vi "Actor Core.vi"(8 "error in":errorcluster, 11 "Launch IMAQ Display in":refnum<class "HIJ Vision Application.lvclass">) -> (0 "error out":errorcluster={"status"=FALSE, "code"=0, "source"="Actor Framework.lvlib:Actor.lvclass:Launch Nested Actor.vi<APPEND>\n\n<b>Complete call chain:</b>\r\n     Actor Framework.lvlib:Actor.lvclass:Launch Nested Actor.vi\r\n     Launch HIJ FileViewer.lvlib:Launch File Viewer.lvclass:Actor Core.vi"}, 3 "Actor out":refnum<class "Actor.lvclass">)   [LabVIEW 2014, in "HIJ Vision Application.lvlib" / "HIJ Vision Application.lvclass"]
doc: "(<B>Filename</B>: Actor Framework.lvlib:Actor.lvclass:Actor Core.vi)\n\nReceives messages to the actor, reacts to them, and initiates any error handling that may shut the actor down.\n\nDescendant classes may override this VI to append parallel tasks for the actor to complete while it handles messages. Overrides use the Call Parent Method node."
uses:
  HIJ Vision Application.lvclass
  <vilib>/ActorFramework/Actor/Actor.lvclass
  <vilib>/ActorFramework/Message Enqueuer/Message Priority.ctl
  HIJ Vision Application Messages/New Results Msg/New Results Msg.lvclass
  HIJ Vision Application.lvclass/HIJ Vision Application.ctl
  Display Actors/HIJ Vision Display/HIJ Vision Display/HIJ Vision Display.lvclass/HIJ Vision Display.ctl
  Analyze/Analyze Actor/Analyze Actor/Analyze Actor.lvclass/Analyze Actor.ctl
  <vilib>/ActorFramework/Actor/Actor.lvclass/Actor.ctl
  <vilib>/ActorFramework/Message Enqueuer/Message Enqueuer.lvclass/Message Enqueuer.ctl
  Display Actors/HIJ Vision Display/HIJ Vision Display Messages/Write Analyze Actor Msg/Write Analyze Enq Msg.lvclass/Write Analyze Enq Msg.ctl
  Shared Code/Viewable Actor/ViewableActor Messages/Insert Into SubPanel Msg/Insert Into SubPanel Msg.lvclass/Insert Into SubPanel Msg.ctl
  Display Actors/HIJ Vision Display/HIJ Vision Display/Read My New Results Msg.vi
  Display Actors/HIJ Vision Display/HIJ Vision Display/Write Publish Analyze Results Msg.vi
  Analyze/Analyze Actor/Analyze Actor/Write Analyze Objects.vi
  Analyze/Analyze Actor/Analyze Actor/Write Publish Analyze Results Msg.vi
  Analyze/Analyze Actor/Analyze Actor/Write Destination.vi
  <vilib>/ActorFramework/Message Enqueuer/Init from Existing Queue.vi
  <vilib>/ActorFramework/Message Enqueuer/Enqueue.vi
  <vilib>/ActorFramework/Message Priority Queue/Priority Enqueue.vi
  Display Actors/HIJ Vision Display/HIJ Vision Display Messages/New Results Msg/New Results Msg.lvclass
  <vilib>/ActorFramework/Message Enqueuer/Message Enqueuer.lvclass
  HIJ Vision Application Messages/After Launch Init Msg/After Launch Init Msg.lvclass
  Display Actors/HIJ Vision Display/HIJ Vision Display Messages/Write Analyze Actor Msg/Write Analyze Enq Msg.lvclass
  Shared Code/Viewable Actor/ViewableActor Messages/Insert Into SubPanel Msg/Insert Into SubPanel Msg.lvclass
  Shared Code/Viewable Actor/ViewableActor/ViewableActor.lvclass
  Display Actors/HIJ Vision Display/HIJ Vision Display/HIJ Vision Display.lvclass
  Analyze/Analyze Actor/Analyze Actor/Analyze Actor.lvclass
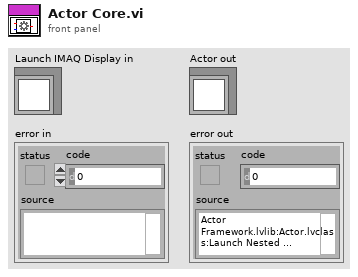
[diagram p1: front panel]
types:
  T1 = typedef "Actor Framework.lvlib/Message Enqueuer.lvclass/Message Priority.ctl" = enum16{"Low", "Normal", "High"}
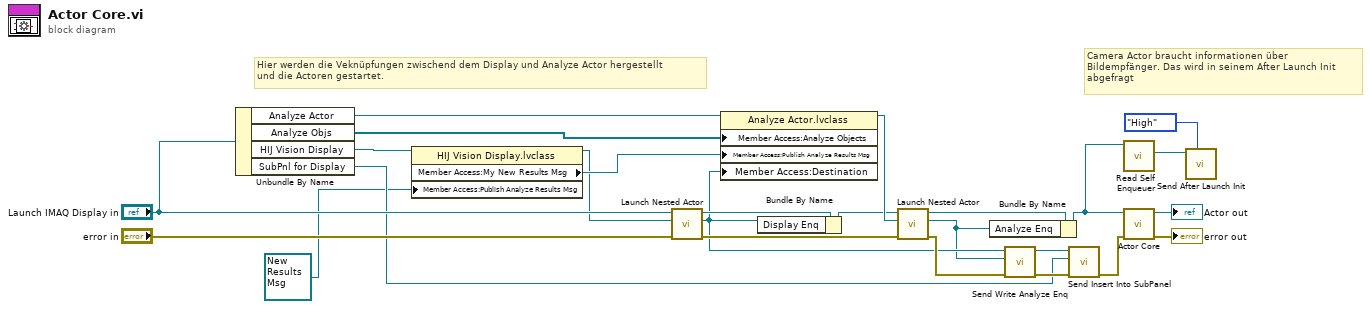
[diagram p0: block diagram]
diagram:
  # "Camera Actor braucht informationen über\nBildempfänger. Das wird in seinem After Launch Init\nabgefragt"
  # "Hier werden die Veknüpfungen zwischend dem Display und Analyze Actor hergestellt\nund die Actoren gestartet."
  n1 = Unbundle By Name("Launch IMAQ Display in") -> ("Analyze Actor"=w13:refnum<class "Analyze Actor.lvclass">, "Analyze Objs"=w14:refnum<class "Analyze BaseClass.lvclass">[], "HIJ Vision Display"=w12:refnum<class "HIJ Vision Display.lvclass">, "SubPnl for Display"=w9:refnum<vi>)
  n2 = property class="HIJ Vision Display.lvclass"(reference=w12, "Member Access:Publish Analyze Results Msg"=refnum<class "New Results Msg.lvclass"> refnum ("HIJ Vision Application.lvlib:New Results Msg.lvclass")) -> (reference out=w10:refnum<class "HIJ Vision Display.lvclass">, "Member Access:My New Results Msg"=w11:refnum<class "New Results Msg.lvclass">)  [unwired: 1 in, 1 out]
  n3 = call <vilib>:"Launch Nested Actor.vi"("error in (no error)"="error in", "Nested Actor"=w10, "Caller Actor in"="Launch IMAQ Display in") -> ("error out"=w22:errorcluster, "Nested Actor's Enqueuer"=w4:refnum<class "Message Enqueuer.lvclass">, "Caller Actor out"=w21:refnum<class "HIJ Vision Application.lvclass">)  [unwired: 6 in]
  n4 = property class="Analyze Actor.lvclass"(reference=w13, "Member Access:Analyze Objects"=w14, "Member Access:Publish Analyze Results Msg"=w11, "Member Access:Destination"=w4) -> (reference out=w20:refnum<class "Analyze Actor.lvclass">)  [unwired: 1 in, 1 out]
  n5 = Bundle By Name(cluster=w21, "Display Enq"=w4) -> (w5:refnum<class "HIJ Vision Application.lvclass">)
  n6 = call <vilib>:"Launch Nested Actor.vi"("error in (no error)"=w22, "Nested Actor"=w20, "Caller Actor in"=w5) -> ("error out"=w18:errorcluster, "Nested Actor's Enqueuer"=w1:refnum<class "Message Enqueuer.lvclass">, "Caller Actor out"=w8:refnum<class "HIJ Vision Application.lvclass">)  [unwired: 6 in]
  n7 = Bundle By Name(cluster=w8, "Analyze Enq"=w1) -> (w2:refnum<class "HIJ Vision Application.lvclass">)
  n8 = call "Send Write Analyze Enq.vi"("error in (no error)"=w18, "Actor Framework:Message Enqueuer"=w1, "Message Enqueuer"=w4) -> ("error out"=w17:errorcluster, "Message Enqueuer out"=w19:refnum<class "Message Enqueuer.lvclass">)  [unwired: 7 in]
  n9 = call "Send Insert Into SubPanel.vi"("error in (no error)"=w17, "SubPanel Ref"=w9, "Message Enqueuer"=w19) -> ("error out"=w16:errorcluster)  [unwired: 7 in, 1 out]
  n10 = call <vilib>:"Read Self Enqueuer.vi"("Actor"=w2) -> ("Self Enqueuer"=w7:refnum<class "Message Enqueuer.lvclass">)  [unwired: 10 in]
  n11 = call-parent "Actor Core.vi"("error in"=w16, "Actor in"=w2) -> ("error out"=→"error out":errorcluster, "Actor out"=→"Actor out":refnum<class "Actor.lvclass">)  [unwired: 8 in]
  n12 = call "Send After Launch Init.vi"("Message Priority (Normal)"=Message_Priority."High", "Message Enqueuer"=w7) -> ()  [unwired: 8 in, 2 out]
